vi "Scan_Ablation_Burst_FindFocus_HighResIntegral_CC.vi"(0 "Offset X-Axis":sgl=30.3, 2 "Offset Y-Axis":sgl=4.5, 3 "X-Axis":sgl=0.1, 5 "Y-Axis":sgl, 8 "Step Size (mm)":sgl=0.01, 9 "ProFile Path":path=path "C:/Users/msg-synapt/Documents/Doktorat/ProFileCSVs/2019/test.csv", 10 "#Pulses":string="5", 11 "Energy":i16(slide)=100 min=0 max=100 step=1 scale=0.0..100.0, 12 "Profile HighRes":string="C:\\Users\\msg-synapt\\Documents\\Doktorat\\ProFileCSVs\\2019\\August\\HR_align", 14 "Offset\n X-Axis 2":sgl, 15 "Offset \nY-Axis 2":sgl, 16 "X-Axis 2":sgl, 17 "Y-Axis 2":sgl, 18 "Step Size in mm 2":sgl=0.01, 19 "Repeats":i32) -> ()   [LabVIEW 2016]
uses:
  <vilib>/DAQmx/write.llb/DAQmx Write (Analog DBL 1Chan 1Samp).vi
  Utility/Global Constants.vi
  Utility/Global_Laser.vi
  <vilib>/DAQmx/create/channels.llb/DAQmx Create Channel (AO-Voltage-Basic).vi
  <vilib>/DAQmx/miscellaneous.llb/DAQmx Fill In Error Info.vi
panel:
  out "CC_send":bool
  in  "z-step":sgl
  in  "z-offset":sgl=0.3
  in  "B-Axis":refnum<k7>(container)
  out "Lambda":dbl
  out "Current Y-Step":i32
  out "Current X-Step":i32
  out "Status?":bool
  out "Abort in \nProgress":bool
  in  "Abort!":bool
  in  "Z-Axis":refnum<k7>(container)
  in  "Y-Axis":refnum<k7>(container)
  in  "X-Axis":refnum<k7>(container)
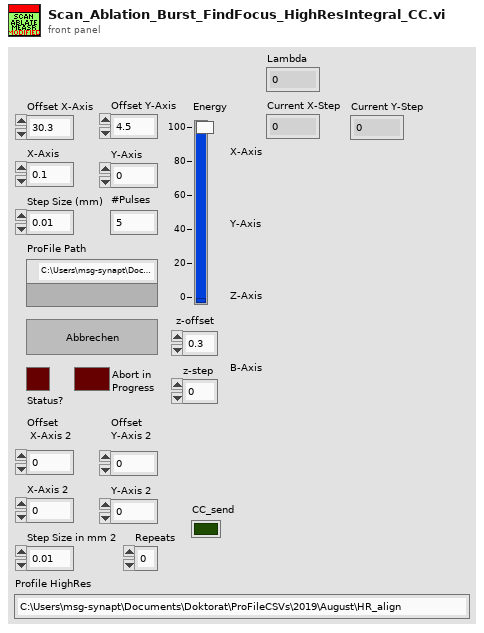
[diagram p1: front panel]
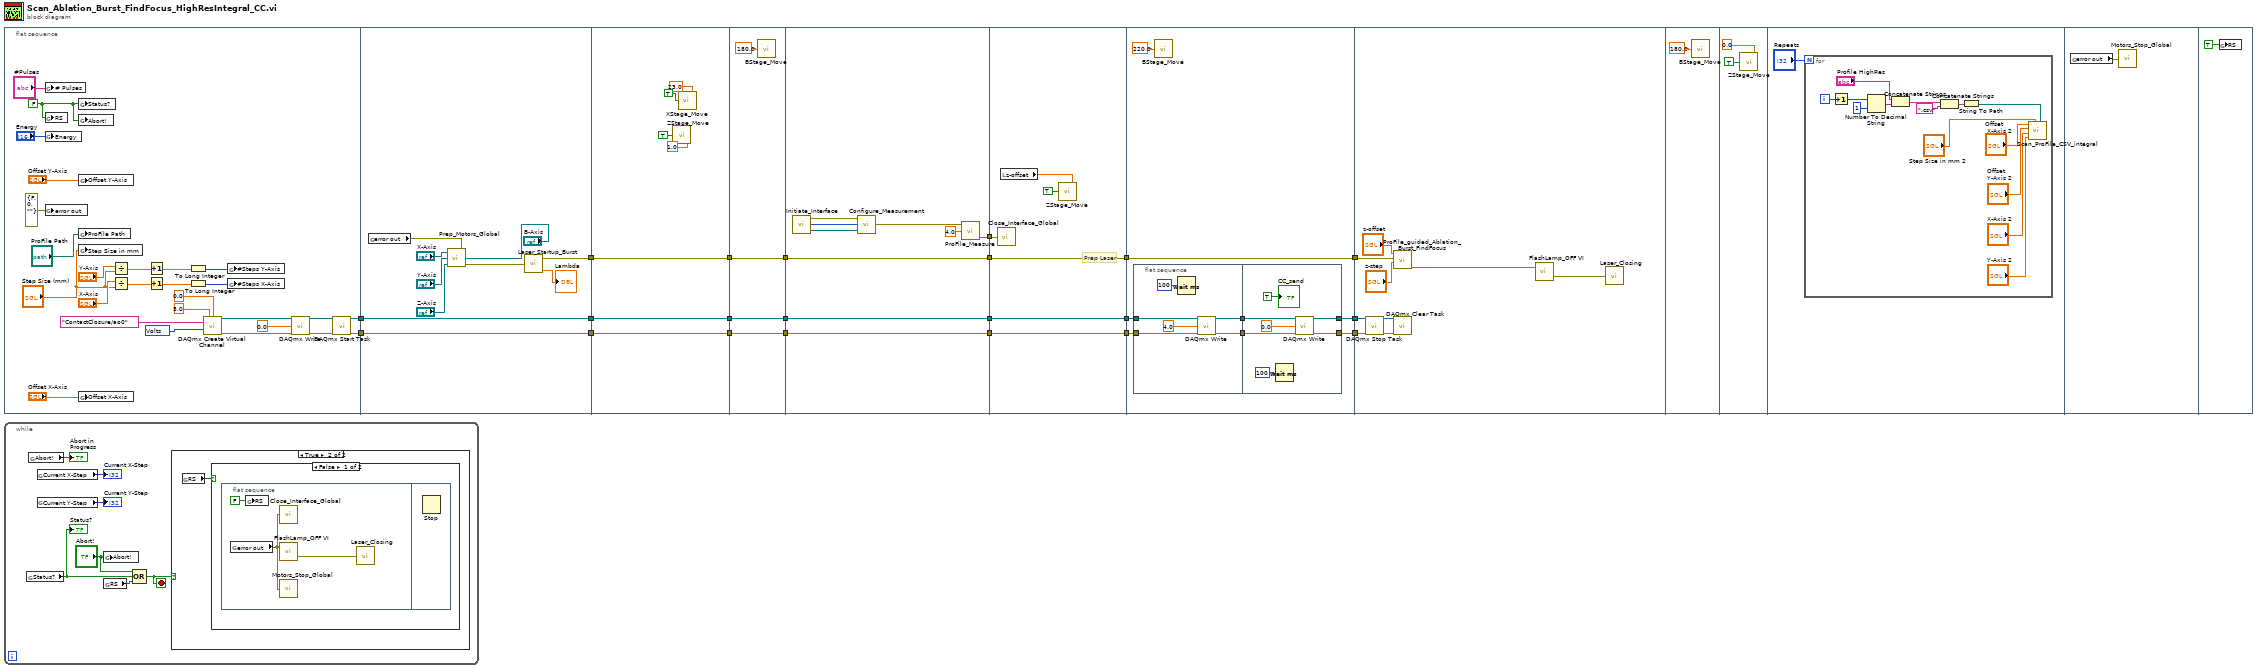
[diagram p0: block diagram]
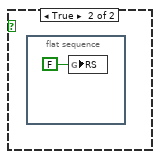
[diagram p3: hidden frame]
diagram:
  n1 = flat-sequence "Flache Sequenzstruktur" {
    tunnel: [w23] -> w16
    tunnel: [w22] -> w12
    tunnel: [w51] -> w6
    tunnel: w16 -> [w50]
    tunnel: [w50] -> w4
    tunnel: w12 -> [w49]
    tunnel: [w49] -> w2
    tunnel: w6 -> [w65]
    tunnel: [w65] -> w5
    tunnel: w4 -> [w64]
    tunnel: [w64] -> w3
    tunnel: w2 -> [w63]
    tunnel: [w63] -> w1
    tunnel: [w68] -> w17
    tunnel: w5 -> [w68]
    tunnel: w3 -> [w67]
    tunnel: [w67] -> w15
    tunnel: [w66] -> w11
    tunnel: w1 -> [w66]
    tunnel: [w78] -> w21
    tunnel: [w73] -> w18
    tunnel: w17 -> [w73]
    tunnel: w15 -> [w71]
    tunnel: [w71] -> w13
    tunnel: w11 -> [w70]
    tunnel: [w70] -> w9
    tunnel: w21 -> [w84]
    tunnel: [w83] -> w20
    tunnel: w18 -> [w83]
    tunnel: [w80] -> w14
    tunnel: w13 -> [w80]
    tunnel: [w79] -> w10
    tunnel: w9 -> [w79]
    tunnel: w20 -> [w92]
    tunnel: [w92] -> w19
    tunnel: w14 -> [w88]
    tunnel: w10 -> [w87]
    tunnel: [w86] -> w8
    tunnel: [w85] -> w7
    tunnel: w19 -> [w114]
    tunnel: w8 -> [w107]
    tunnel: w7 -> [w106]
    frame #0 {
      w26 = 10348 items=["Volts"=10348, "From Custom Scale"=10065] ("units")
      w33 = FALSE
      n2 = global write "Global_Laser.vi" "# Pulses"("#Pulses") -> ()
      n3 = global write "Global Constants.vi" "RS"(w33) -> ()
      n4 = global write "Global_Laser.vi" "Energy"("Energy") -> ()
      n5 = global write "Global Constants.vi" "error out"(errorcluster {"status"=FALSE, "code"=0, "source"=""} ("error")) -> ()
      n6 = global write "Global Constants.vi" "Status?"(w33) -> ()
      n7 = global write "Global Constants.vi" "Abort!"(w33) -> ()
      n8 = global write "Global Constants.vi" "Offset Y-Axis"("Offset Y-Axis") -> ()
      n9 = global write "Global Constants.vi" "ProFile Path"("ProFile Path") -> ()
      n10 = global write "Global Constants.vi" "Step Size in mm"("Step Size (mm)") -> ()
      n11 = global write "Global Constants.vi" "Offset X-Axis"("Offset X-Axis") -> ()
      n12 = Divide(x="Y-Axis", y="Step Size (mm)") -> (x/y=w46:sgl)
      n13 = Divide(x="X-Axis", y="Step Size (mm)") -> (x/y=w45:sgl)
      n14 = Increment(x=w46) -> (x+1=w48:sgl)
      n15 = Increment(x=w45) -> (x+1=w47:sgl)
      n16 = To Long Integer(number=w48) -> (32bit integer=w43:i32)
      n17 = To Long Integer(number=w47) -> (32bit integer=w44:i32)
      n18 = call-poly <vilib>:"DAQmx Create Virtual Channel.vi"("maximum value"=5.0, "minimum value"=0.0, "physical channels"=tag "ContactClosure/ao0", "units"=w26) -> ("task out"=w30:refnum<k21>, "error out"=w32:errorcluster)  [unwired: 10 in]
      n19 = global write "Global Constants.vi" "#Steps Y-Axis"(w43) -> ()
      n20 = global write "Global Constants.vi" "#Steps X-Axis"(w44) -> ()
      n21 = call-poly <vilib>:"DAQmx Write.vi"("task/channels in"=w30, "data"=0.0, "error in"=w32) -> ("task out"=w29:refnum<k21>, "error out"=w31:errorcluster)  [unwired: 10 in, 1 out]
      n22 = call <vilib>:"DAQmx Start Task.vi"("task/channels in"=w29, "error in"=w31) -> ("task out"=w23:refnum<k21>, "error out"=w22:errorcluster)  [unwired: 12 in]
    }
    frame #1 {
      n23 = global read "Global Constants.vi" "error out"() -> (w55:errorcluster)
      n24 = call "Prep_Motors_Global.vi"("B-Axis"="B-Axis", "Error In"=w55, "Z-Axis"="Z-Axis", "Y-Axis"="Y-Axis", "X-Axis"="X-Axis") -> ("Error Out"=w52:errorcluster)
      n25 = call "Laser_Startup_Burst.vi"("Error In"=w52) -> ("Lambda"=→"Lambda":dbl, "Error Out"=w51:errorcluster)
    }
    frame #2 {
      n26 = call "ZStage_Move.vi"("Position"=sgl 1.0, "Z_Wait"=TRUE) -> ()
      n27 = call "XStage_Move.vi"("Position"=sgl 23.0, "X_Wait"=TRUE) -> ()
    }
    frame #3 {
      n28 = call "BStage_Move.vi"("Position"=sgl 180.0) -> ()
    }
    frame #4 {
      n29 = call "Initiate_Interface.vi"() -> ("DLL-Path"=w77:path, "instanceHandle"=w76:u32, "Fehler (Ausgang)"=w75:errorcluster)
      n30 = call "Configure_Measurement.vi"("DLL-Path"=w77, "instanceHandle"=w76, "Error In"=w75) -> ("Fehler (Ausgang)"=w74:errorcluster)
      n31 = call "ProFile_Measure.vi"("Ceiling"=sgl 4.0, "error in"=w74) -> ("error out"=w78:errorcluster)
    }
    frame #5 {
      # "Prep Laser"
      n32 = call "Close_Interface_Global.vi"("Error In"=w84) -> ()
      n33 = local read "z-offset"() -> (w81:sgl)
      n34 = call "ZStage_Move.vi"("Position"=w81, "Z_Wait"=TRUE) -> ()
    }
    frame #6 {
      n35 = flat-sequence {
        tunnel: [w98] -> w89
        tunnel: [w97] -> w90
        tunnel: w88 -> [w94]
        tunnel: w87 -> [w93]
        tunnel: [w100] -> w86
        tunnel: [w101] -> w85
        tunnel: w90 -> [w104]
        tunnel: w89 -> [w105]
        frame #0 {
          n36 = Wait (ms)(milliseconds to wait=u32 100) -> ()  [unwired: 1 out]
          n37 = call-poly <vilib>:"DAQmx Write.vi"("task/channels in"=w94, "data"=4.0, "error in"=w93) -> ("task out"=w98:refnum<k21>, "error out"=w97:errorcluster)  [unwired: 10 in, 1 out]
        }
        frame #1 {
          n38 = Wait (ms)(milliseconds to wait=u32 100) -> ()  [unwired: 1 out]
          n39 = call-poly <vilib>:"DAQmx Write.vi"("task/channels in"=w105, "data"=0.0, "error in"=w104) -> ("task out"=w101:refnum<k21>, "error out"=w100:errorcluster)  [unwired: 10 in, 1 out]
          "CC_send" <- TRUE ("CC_send")
        }
      }
      n40 = call "BStage_Move.vi"("Position"=sgl 220.0) -> ()
    }
    frame #7 {
      n41 = call <vilib>:"DAQmx Stop Task.vi"("task/channels in"=w106, "error in"=w107) -> ("task out"=w109:refnum<k21>, "error out"=w108:errorcluster)  [unwired: 12 in]
      n42 = call "ProFile_guided_Ablation_Burst_FindFocus.vi"("z-step"="z-step", "Error In"=w114, "z-offset"="z-offset") -> ("error out"=w112:errorcluster)
      n43 = call <vilib>:"DAQmx Clear Task.vi"("task in"=w109, "error in"=w108) -> ()  [unwired: 13 in, 1 out]
      n44 = call "FlashLamp_OFF VI.vi"("Error In"=w112) -> ("error out"=w113:errorcluster)
      n45 = call "Laser_Closing.vi"("Error In"=w113) -> ()
    }
    frame #8 {
      n46 = call "BStage_Move.vi"("Position"=sgl 180.0) -> ()
    }
    frame #9 {
      n47 = call "ZStage_Move.vi"("Position"=sgl 0.0, "Z_Wait"=TRUE) -> ()
    }
    frame #10 {
      n48 = for {
        N: "Repeats" -> [_]
        i -> [w124]
        n49 = Increment(x=w124) -> (x+1=w123:i32)
        n50 = Number To Decimal String(number=w123, width (-)=i16 1 ("Breite (-)")) -> (decimal integer string=w122:string)
        n51 = Concatenate Strings("Profile HighRes", w122) -> (w121:string)
        n52 = Concatenate Strings(w121, ".csv" ("String")) -> (w119:string)
        n53 = String To Path(string=w119) -> (path=w127:path)
        n54 = call "Scan_ProFile_CSV_integral.vi"("ProFile Path"=w127, "Step Size in mm"="Step Size in mm 2", "Y-Axis"="Y-Axis 2", "X-Axis"="X-Axis 2", "Offset Y-Axis"="Offset \nY-Axis 2", "Offset X-Axis"="Offset\n X-Axis 2") -> ()  [unwired: 6 in]
      }
    }
    frame #11 {
      n55 = global read "Global Constants.vi" "error out"() -> (w133:errorcluster)
      n56 = call "Motors_Stop_Global.vi"("error in"=w133) -> ()
    }
    frame #12 {
      n57 = global write "Global Constants.vi" "RS"(TRUE) -> ()
    }
  }
  n58 = while {
    stop <- w140 stop-if-true
    n59 = global read "Global Constants.vi" "Status?"() -> (w136:bool)
    "Status?" <- w136
    n60 = global read "Global Constants.vi" "Abort!"() -> (→"Abort in \nProgress":bool)
    n61 = global read "Global Constants.vi" "Current X-Step"() -> (→"Current X-Step":i32)
    n62 = global read "Global Constants.vi" "Current Y-Step"() -> (→"Current Y-Step":i32)
    n63 = global write "Global Constants.vi" "Abort!"("Abort!") -> ()
    n64 = global read "Global Constants.vi" "RS"() -> (w135:bool)
    n65 = Compound Arithmetic op=OR("Abort!", w136, w135) -> (w140:bool)
    n66 = case shown="True" w140 {
      frame False {
      }
      frame True {
        n67 = global read "Global Constants.vi" "RS"() -> (w142:bool)
        n68 = case shown="False" w142 {
          frame False {
            n69 = flat-sequence {
              frame #0 {
                n70 = global read "Global Constants.vi" "error out"() -> (w144:errorcluster)
                n71 = global write "Global Constants.vi" "RS"(FALSE) -> ()
                n72 = call "Close_Interface_Global.vi"("Error In"=w144) -> ()
                n73 = call "FlashLamp_OFF VI.vi"("Error In"=w144) -> ("error out"=w145:errorcluster)
                n74 = call "Motors_Stop_Global.vi"("error in"=w144) -> ()
                n75 = call "Laser_Closing.vi"("Error In"=w145) -> ()
              }
              frame #1 {
                n76 = Stop() -> ()  [unwired: 1 in]
              }
            }
          }
          frame True {
            n77 = flat-sequence {
              frame #0 {
                n78 = global write "Global Constants.vi" "RS"(FALSE) -> ()
              }
            }
          }
        }
      }
    }
  }
